vi "get_image_offset.vi"(8 "error in (no error)":errorcluster, 11 "TrajectoryDL110420DoubleCircle in":refnum<class "TrajectoryDL110420DoubleCircle.lvclass">) -> (0 "error out":errorcluster, 2 "offset":refnum<class "SpaceVector.lvclass">, 3 "TrajectoryDL110420DoubleCircle out":refnum<class "TrajectoryDL110420DoubleCircle.lvclass">)   [LabVIEW 2010, in "TrajectoryDL110420DoubleCircle.lvclass"]
uses:
  TrajectoryDL110420DoubleCircle.lvclass
  common/classes/SpaceVector/SpaceVector/SpaceVector.lvclass
  TrajectoryDL110420DoubleCircle.lvclass/TrajectoryDL110420DoubleCircle.ctl
  common/classes/XMLElement/XMLElement/XMLElement.lvclass
  common/classes/ImageCollection/ImageCollection/ImageCollection.lvclass
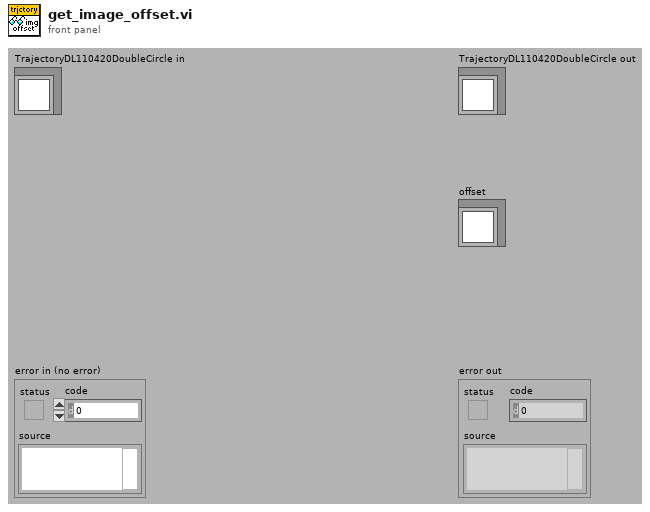
[diagram p1: front panel]
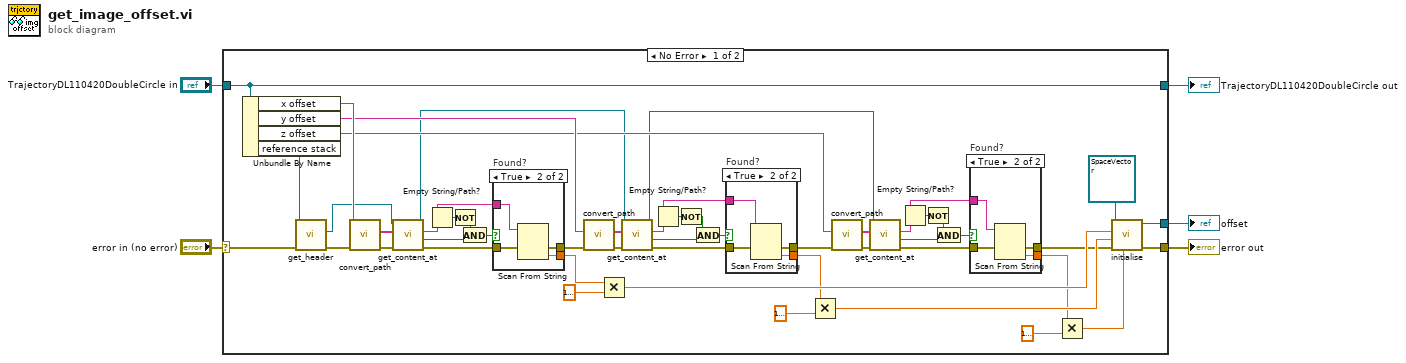
[diagram p0: block diagram]
diagram:
  n1 = case shown="No Error" "error in (no error)" {
    selector: "error in (no error)" -> [w24 w71]
    tunnel: [w45 w71] -> w4
    tunnel: [w54 w70] -> w2
    tunnel: "TrajectoryDL110420DoubleCircle in" -> [w54 w70]
    tunnel: [w44 _] -> w1
    frame No Error {
      n2 = Unbundle By Name(w54) -> ("x offset"=w51:string, "y offset"=w37:string, "z offset"=w31:string, "reference stack"=w23:refnum<class "ImageCollection.lvclass">)
      n3 = call "get_header.vi"("error in (no error)"=w24, "ImageCollection in"=w23) -> ("error out"=w21:errorcluster, "header"=w22:refnum<class "XMLElement.lvclass">)  [unwired: 7 in, 1 out]
      n4 = call "convert_path.vi"("error in (no error)"=w21, "xpath in"=w51) -> ("error out"=w53:errorcluster, "key array out"=w52:string[])  [unwired: 7 in, 1 out]
      n5 = call "get_content_at.vi"("error in (no error)"=w53, "key chain"=w52, "Element in"=w22) -> ("error out"=w50:errorcluster, "found?"=w17:bool, "string"=w20:string, "Element out"=w26:refnum<class "XMLElement.lvclass">)  [unwired: 5 in]
      n6 = Empty String/Path?(string/path=w20) -> (empty?=w19:bool)
      n7 = Not(x=w19) -> (.not. x?=w18:bool)
      n8 = And(x=w18, y=w17) -> (x .and. y?=w16:bool)
      n9 = case "Found?" shown="True" w16 {
        tunnel: w50 -> [w65 w69]
        tunnel: [w65 w68] -> w46
        tunnel: w20 -> [_ w67]
        tunnel: [_ w66] -> w43
        frame False {
        }
        frame True {
          n10 = Scan From String(input string=w67, error in=w69) -> (error out=w68:errorcluster, output 1=w66:dbl)  [unwired: 3 in, 2 out]
        }
      }
      n11 = call "convert_path.vi"("error in (no error)"=w46, "xpath in"=w37) -> ("error out"=w47:errorcluster, "key array out"=w48:string[])  [unwired: 7 in, 1 out]
      n12 = Multiply(x=w43, y=dbl[unit] 1e-06) -> (x*y=w41:dbl[unit])
      n13 = call "get_content_at.vi"("error in (no error)"=w47, "key chain"=w48, "Element in"=w26) -> ("error out"=w49:errorcluster, "found?"=w7:bool, "string"=w8:string, "Element out"=w25:refnum<class "XMLElement.lvclass">)  [unwired: 5 in]
      n14 = Empty String/Path?(string/path=w8) -> (empty?=w14:bool)
      n15 = Not(x=w14) -> (.not. x?=w15:bool)
      n16 = And(x=w15, y=w7) -> (x .and. y?=w6:bool)
      n17 = case "Found?" shown="True" w6 {
        tunnel: w49 -> [w60 w64]
        tunnel: [w60 w63] -> w32
        tunnel: w8 -> [_ w62]
        tunnel: [_ w61] -> w39
        frame False {
        }
        frame True {
          n18 = Scan From String(input string=w62, error in=w64) -> (error out=w63:errorcluster, output 1=w61:dbl)  [unwired: 3 in, 2 out]
        }
      }
      n19 = Multiply(x=w39, y=dbl[unit] 1e-06) -> (x*y=w38:dbl[unit])
      n20 = call "convert_path.vi"("error in (no error)"=w32, "xpath in"=w31) -> ("error out"=w36:errorcluster, "key array out"=w35:string[])  [unwired: 7 in, 1 out]
      n21 = call "get_content_at.vi"("error in (no error)"=w36, "key chain"=w35, "Element in"=w25) -> ("error out"=w34:errorcluster, "found?"=w10:bool, "string"=w11:string)  [unwired: 5 in, 1 out]
      n22 = Empty String/Path?(string/path=w11) -> (empty?=w13:bool)
      n23 = Not(x=w13) -> (.not. x?=w12:bool)
      n24 = And(x=w12, y=w10) -> (x .and. y?=w9:bool)
      n25 = case "Found?" shown="True" w9 {
        tunnel: w34 -> [w55 w59]
        tunnel: [w55 w58] -> w33
        tunnel: w11 -> [_ w57]
        tunnel: [_ w56] -> w29
        frame False {
        }
        frame True {
          n26 = Scan From String(input string=w57, error in=w59) -> (error out=w58:errorcluster, output 1=w56:dbl)  [unwired: 3 in, 2 out]
        }
      }
      n27 = Multiply(x=w29, y=dbl[unit] 1e-06) -> (x*y=w28:dbl[unit])
      n28 = call "initialise.vi"("z"=w28, "error in (no error)"=w33, "y"=w38, "x"=w41, "SpaceVector in"=refnum<class "SpaceVector.lvclass"> refnum ("SpaceVector.lvclass")) -> ("error out"=w45:errorcluster, "SpaceVector out"=w44:refnum<class "SpaceVector.lvclass">)  [unwired: 5 in]
    }
    frame Error {
    }
  }
  "error out" <- w4
  "TrajectoryDL110420DoubleCircle out" <- w2
  "offset" <- w1
